vi "send_pilot_scenario.vi"(0 "simx in":T1={"Config"={"Trajectory"={"Number of frames"=0, "Frame number"=0, "Trajectory"=""}, "Weather"={"id"=""}}, "Connections"={"Simulator Connection"=refnum, "server_ip"="127.0.0.1", "Port"=0, "Sensor connections"=[]}, "Map"={"lanes"={"x"=[], "y"=[], "z"=[]}, "StartPosition"={"start_points"={"locations"=[], "rotations"=[], "type"=[]}, "StartRotation"=[], "StartLocation"=[]}, "Draw Map Size"={"Width"=0, "Height"=0}, "DrawArea"={"min_Y"=0.0, "min_X"=0.0, "Scale X"=0.0, "Scale Y"=0.0}, "Map"=bytes[0], "Map Geojson"=""}}, 2 "Scenario Configuration":path, 5 "error in":errorcluster) -> (6 "simx out":T1={"Config"={"Trajectory"={"Number of frames"=0, "Frame number"=0, "Trajectory"=""}, "Weather"={"id"=""}}, "Connections"={"Simulator Connection"=refnum, "server_ip"="127.0.0.1", "Port"=0, "Sensor connections"=[]}, "Map"={"lanes"={"x"=[], "y"=[], "z"=[]}, "StartPosition"={"start_points"={"locations"=[], "rotations"=[], "type"=[]}, "StartRotation"=[], "StartLocation"=[]}, "Draw Map Size"={"Width"=0, "Height"=0}, "DrawArea"={"min_Y"=0.0, "min_X"=0.0, "Scale X"=0.0, "Scale Y"=0.0}, "Map"=bytes[0], "Map Geojson"=""}}, 7 "Scenario configuration":string, 8 "error out":errorcluster)   [LabVIEW 2019, in "Lib_Simx.lvlib"]
doc: "Reads an scenario file and sends it to the server."
uses:
  Lib_Simx.lvlib
  controls/simx_connection.ctl
  controls/config.ctl
  controls/trajectory.ctl
  controls/weather.ctl
  controls/connections.ctl
  controls/start_points.ctl
  <vilib>/Utility/miscctls.llb/LVBoundsTypeDef.ctl
  tools/simx_common.vi
panel:
  out "config response":string
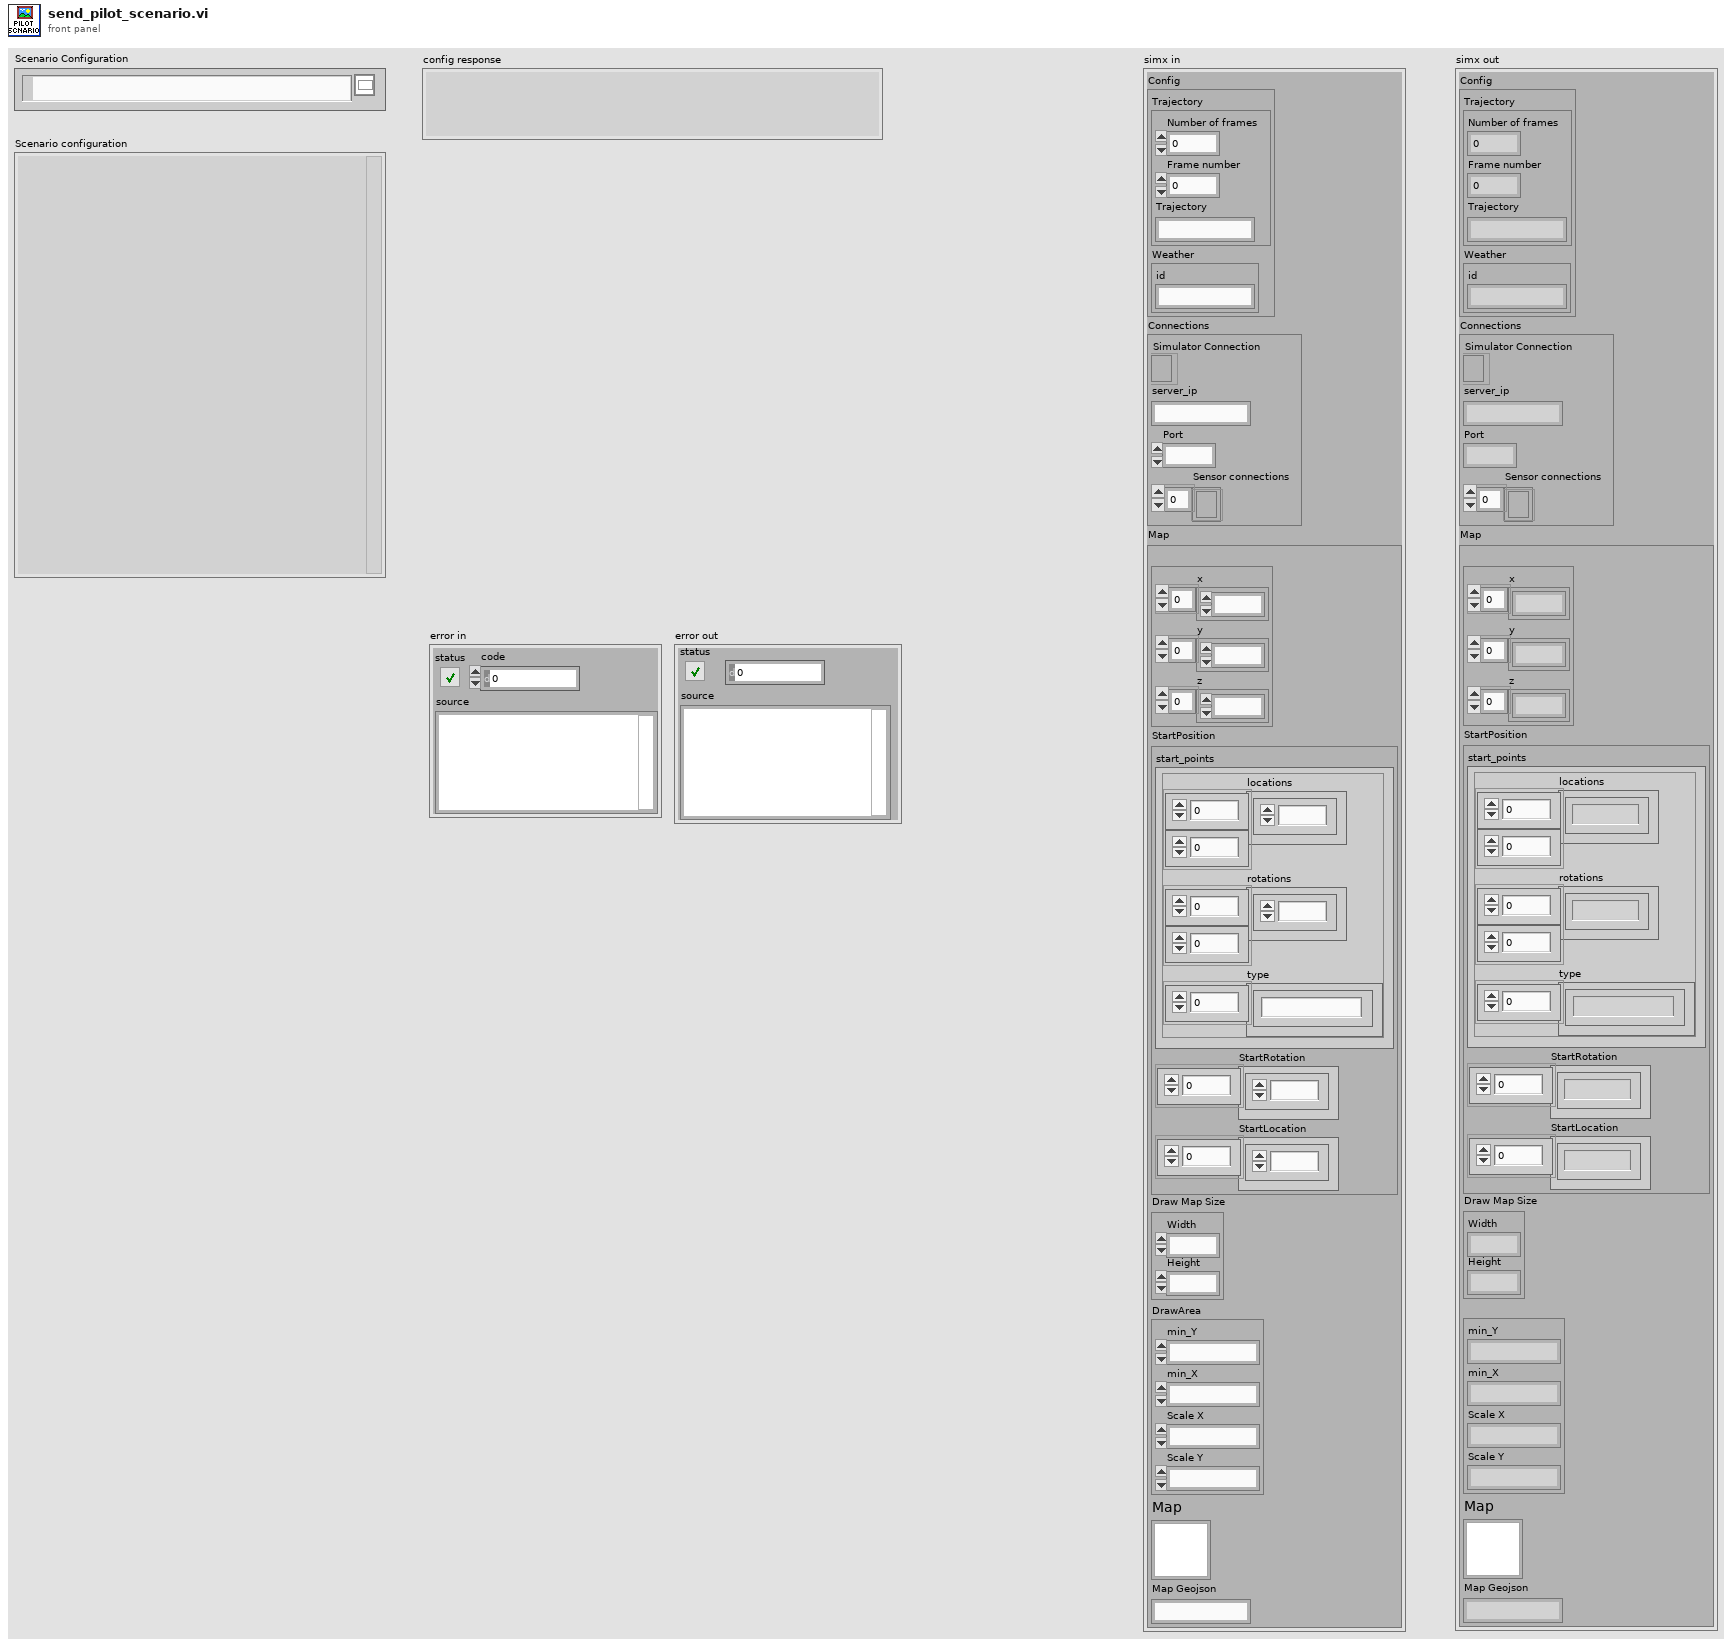
[diagram p1: front panel]
types:
  T1 = typedef "Lib_Simx.lvlib/simx_connection.ctl" = cluster{"Config":T2, "Connections":T5, "Map":cluster{"lanes":cluster{"x":dbl[], "y":dbl[], "z":dbl[]}, "StartPosition":cluster{"start_points":T6, "StartRotation":dbl[], "StartLocation":dbl[]}, "Draw Map Size":T7, "DrawArea":cluster{"min_Y":dbl, "min_X":dbl, "Scale X":dbl, "Scale Y":dbl}, "Map":picture, "Map Geojson":string}}
  T2 = typedef "Lib_Simx.lvlib/config.ctl" = cluster{"Trajectory":T3, "Weather":T4}
  T3 = typedef "Lib_Simx.lvlib/trajectory.ctl" = cluster{"Number of frames":i32, "Frame number":i32, "Trajectory":string}
  T4 = typedef "Lib_Simx.lvlib/weather.ctl" = cluster{"id":string}
  T5 = typedef "Lib_Simx.lvlib/connections.ctl" = cluster{"Simulator Connection":refnum<k5>, "server_ip":string, "Port":i32, "Sensor connections":refnum<k5>[]}
  T6 = typedef "Lib_Simx.lvlib/start_points.ctl" = cluster{"locations":dbl[][], "rotations":dbl[][], "type":string[]}
  T7 = typedef "LVBoundsTypeDef.ctl" = cluster{"Width":u32, "Height":u32}
  T8 = cluster{"vehicles":cluster{"behavior_settings":cluster{"destroy_on_collision":bool, "ignore_lane_change_boxes":bool, "ignore_other_vehicles":bool, "ignore_traffic_signals":bool, "initial_speed_is_delta":bool, "limit_speed_in_curves":bool, "obey_road_speed_limits":bool, "snap_to_lane":bool}, "body_color":string, "class_path":string, "controller_settings":cluster{"delayed_start":i32, "distance_to_stop_sign":i32, "initial_speed":i32, "lane_offset":i32, "rolling_stop_speed":i32, "search_forward_distance":i32, "set_speed":i32, "spawn_offset":cluster{"x":i32, "y":i32, "z":i32}, "steer_forward_distance":cluster{"x":i32, "y":i32}, "steer_forward_distance_lane_change":cluster{"x":i32, "y":i32}, "steer_forward_speed":cluster{"x":i32, "y":i32}, "turn_preference":i32}, "location":cluster{"x":dbl, "y":i32, "z":i32}, "name":string, "rotation":cluster{"pitch":i32, "roll":i32, "yaw":i32}, "scale":cluster{"x":i32, "y":i32, "z":i32}, "tags":string[]}[]}
  T9 = cluster{"behavior_settings":cluster{"destroy_on_collision":bool, "ignore_lane_change_boxes":bool, "ignore_other_vehicles":bool, "ignore_traffic_signals":bool, "initial_speed_is_delta":bool, "limit_speed_in_curves":bool, "obey_road_speed_limits":bool, "snap_to_lane":bool}, "body_color":string, "class_path":string, "controller_settings":cluster{"delayed_start":i32, "distance_to_stop_sign":i32, "initial_speed":i32, "lane_offset":i32, "rolling_stop_speed":i32, "search_forward_distance":i32, "set_speed":i32, "spawn_offset":cluster{"x":i32, "y":i32, "z":i32}, "steer_forward_distance":cluster{"x":i32, "y":i32}, "steer_forward_distance_lane_change":cluster{"x":i32, "y":i32}, "steer_forward_speed":cluster{"x":i32, "y":i32}, "turn_preference":i32}, "location":cluster{"x":dbl, "y":i32, "z":i32}, "name":string, "rotation":cluster{"pitch":i32, "roll":i32, "yaw":i32}, "scale":cluster{"x":i32, "y":i32, "z":i32}, "tags":string[]}[]
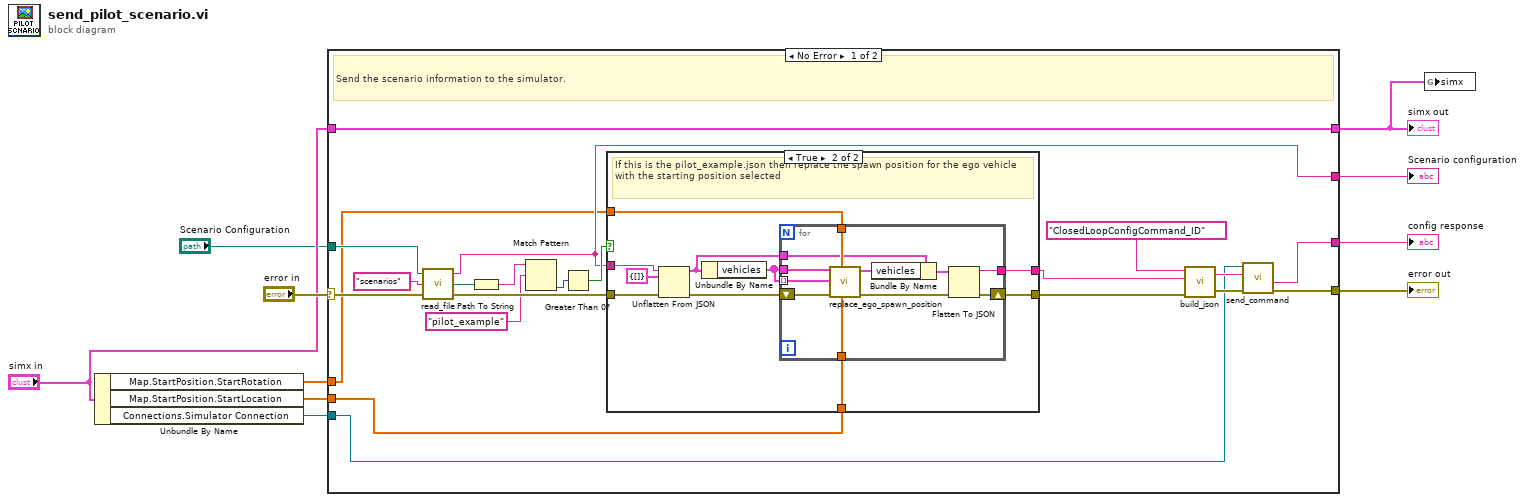
[diagram p0: block diagram]
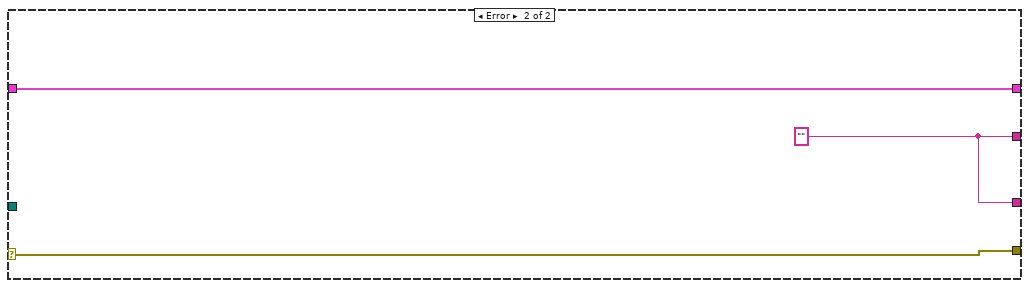
[diagram p3: hidden frame]
diagram:
  n1 = Unbundle By Name("simx in") -> ("Map.StartPosition.StartRotation"=w4:dbl[], "Map.StartPosition.StartLocation"=w3:dbl[], "Connections.Simulator Connection"=w1:refnum<k5>)
  n2 = case shown="No Error" "error in" {
    selector: "error in" -> [w27 w57]
    tunnel: [w31 w55] -> w10
    tunnel: [w30 w57] -> w9
    tunnel: "simx in" -> [w16 w56]
    tunnel: [w16 w56] -> w2
    tunnel: [w18 w55] -> w6
    tunnel: "Scenario Configuration" -> [w23 _]
    tunnel: w4 -> [w13 _]
    tunnel: w3 -> [w14 _]
    tunnel: w1 -> [w12 _]
    frame No Error {
      # "Send the scenario information to the simulator."
      n3 = call "read_file.vi"("error in"=w27, "Base directory name"="scenarios" ("Folder path"), "File path in"=w23) -> ("error out"=w25:errorcluster, "File path out"=w15:path, "Trajectory or Scenario read"=w18:string)
      n4 = Path To String(path=w15) -> (string=w22:string)
      n5 = Match Pattern(string=w22, regular expression="pilot_example") -> (offset past match=w20:i32)  [unwired: 1 in, 3 out]
      n6 = Greater Than 0?(x=w20) -> (x > 0?=w19:bool)
      n7 = case shown="True" w19 {
        tunnel: w18 -> [w33 w43]
        tunnel: [w33 w42] -> w26
        tunnel: w14 -> [_ w40]
        tunnel: w13 -> [_ w41]
        tunnel: w25 -> [w32 w39]
        tunnel: [w32 w37] -> w24
        frame False {
          # "Send the original scenario"
        }
        frame True {
          # "If this is the pilot_example.json then replace the spawn position for the ego vehicle with the starting position selected"
          n8 = Unflatten From JSON(JSON string=w43, type and defaults=T8 {"vehicles"=[]} ("Cluster"), error in (no error)=w39) -> (value=w35:T8, error out=w38:errorcluster)  [unwired: 4 in]
          n9 = Unbundle By Name(w35) -> ("vehicles"=w36:T9)
          n10 = for {
            tunnel: w36 -> [w45] mode=indexing
            tunnel: [w54] -> w42
            tunnel: w41 -> [w53]
            tunnel: w40 -> [w52]
            shift-right: [w51] -> w37
            shift-left: w38 -> [w47]
            tunnel: w36 -> [w50]
            tunnel: w35 -> [w49]
            n11 = call "replace_ego_spawn_position.vi"("Start location"=w52, "Start rotation"=w53, "error in"=w47, "Cluster"=w45, "vehicles"=w50) -> ("error out"=w46:errorcluster, "vehicles out"=w44:T9)  [unwired: 3 in]
            n12 = Bundle By Name(cluster=w49, "vehicles"=w44) -> (w48:T8)
            n13 = Flatten To JSON(anything=w48, error in (no error)=w46) -> (JSON string=w54:string, 11:w51:errorcluster)  [unwired: 1 in]
          }
        }
      }
      n14 = call "build_json.vi"("error in"=w24, "Message"=w26, "Command_ID"="ClosedLoopConfigCommand_ID") -> ("error out"=w28:errorcluster, "JSON Out"=w29:string)  [unwired: 1 in]
      n15 = call "send_command.vi"("error in"=w28, "JSON Command"=w29, "TCP Network Connection in"=w12) -> ("error out"=w30:errorcluster, "Response"=w31:string)  [unwired: 1 in, 2 out]
    }
    frame Error {
      w55 = "" ("response")
    }
  }
  "config response" <- w10
  "error out" <- w9
  "simx out" <- w2
  "Scenario configuration" <- w6
  n16 = global write "simx_common.vi" "simx"(w2) -> ()
